vi "search-label.vi"(10 "label":string, 11 "command-stack":string[](array[string])) -> (2 "Numeric":i32, 3 "Boolean":bool)   [LabVIEW 2017]
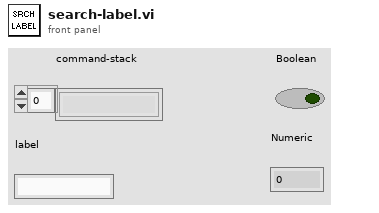
[diagram p1: front panel]
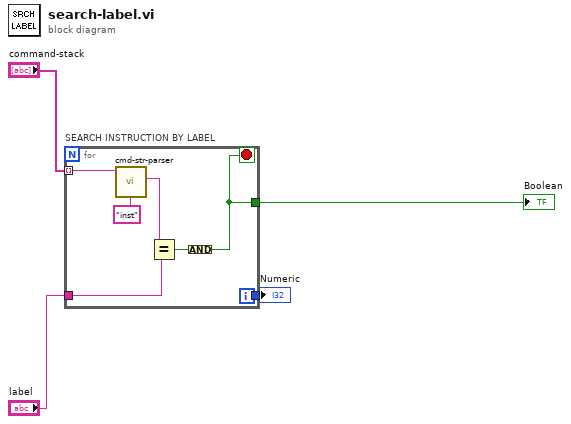
[diagram p0: block diagram]
diagram:
  n1 = for "SEARCH INSTRUCTION BY LABEL" {
    tunnel: "command-stack" -> [w7] mode=indexing
    tunnel: [w11] -> w3
    tunnel: "label" -> [w8]
    tunnel: [w9] -> w2
    i -> [w11]
    stop <- w9 stop-if-true
    n2 = call "cmd-str-parser.vi"("name"="inst", "command in"=w7) -> ("value out"=w6:string)  [unwired: 7 in, 2 out]
    n3 = Equal?(x=w8, y=w6) -> (x = y?=w10:bool)
    n4 = Compound Arithmetic op=AND(w10) -> (w9:bool)
  }
  "Numeric" <- w3
  "Boolean" <- w2
